vi "PCO_SetSoftFPS.vi"(0 "ph":u64, 1 "dwFPSin":u32, 2 "dwExp":u32, 3 "wTimeBaseExp":u16(ring) items=["ns", "us", "ms"], 4 "wFlags":u16, 5 "error in (no error)":errorcluster {"code" format="%x"}) -> (14 "ph_out":u64, 15 "ErrorMessage":i32 format="%x", 16 "dwFPSout":u32, 18 "wFlagsOut":u16, 19 "error out":errorcluster {"code" format="%x"})   [LabVIEW 2019, in "SDK.lvlib" / "TimingControl.lvlib"]
doc: "Setss the timing for the specified FPS (frames per second). The FPS is set by running an iterative loop, so reponse time may be slow."
uses:
  TimingControl.lvlib
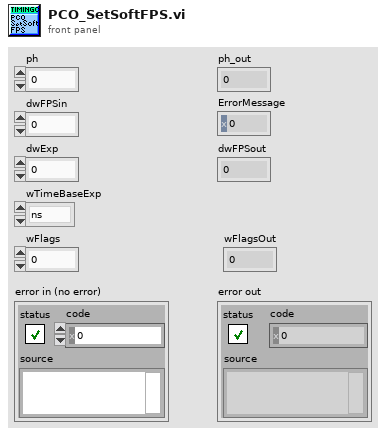
[diagram p1: front panel]
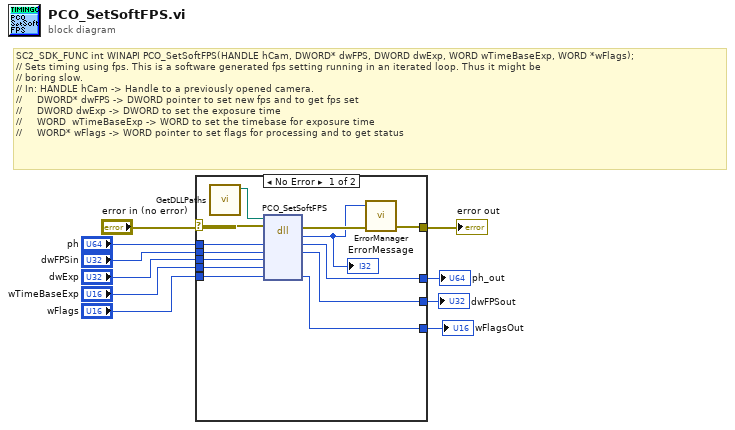
[diagram p0: block diagram]
diagram:
  # "SC2_SDK_FUNC int WINAPI PCO_SetSoftFPS(HANDLE hCam, DWORD* dwFPS, DWORD dwExp, WORD wTimeBaseExp, WORD *wFlags);\n// Sets timing using fps. This is a software generated fps setting running in an iterated loop. Thus it might be\n// boring slow.\n// In: HANDLE hCam -> Handle to a previously opened camera.\n//     DWORD* dwFPS -> DWORD pointer to set new fps and to get fps set\n//     DWORD dwExp -> DWORD to set the exposure time\n//     WORD  wTimeBaseExp -> WORD to set the timebase for exposure time\n//     WORD* wFlags -> WORD pointer to set flags for processing and to get status"
  n1 = case shown="No Error" "error in (no error)" {
    selector: "error in (no error)" -> [w21 w27]
    tunnel: "ph" -> [w23 w26]
    tunnel: "dwFPSin" -> [w22 w25]
    tunnel: [w19 w27] -> w9
    tunnel: [w16 w26] -> w7
    tunnel: [w15 w25] -> w6
    tunnel: "dwExp" -> [w14 _]
    tunnel: "wTimeBaseExp" -> [w13 _]
    tunnel: "wFlags" -> [w12 w24]
    tunnel: [w11 w24] -> w1
    frame No Error {
      n2 = call "GetDLLPaths.vi"() -> ("SC2_Cam_Path"=w17:path)  [unwired: 8 in, 3 out]
      n3 = dll-call lib="?" fn="PCO_SetSoftFPS"(path in=w17, error in=w21, "ph"=w23, "dwFPS"=w22, "dwExp"=w14, "wTimeBaseExp"=w13, "wFlags"=w12) -> (error out=w20:errorcluster, "return type"=w18:i32, "ph"=w16:u64, "dwFPS"=w15:u32, "wFlags"=w11:u16)  [unwired: 3 in, 1 out]
      "ErrorMessage" <- w18
      n4 = call "ErrorManager.vi"("error in (no error)"=w20, "error code"=w18) -> ("error out"=w19:errorcluster)  [unwired: 2 in, 1 out]
    }
    frame Error {
    }
  }
  "error out" <- w9
  "ph_out" <- w7
  "dwFPSout" <- w6
  "wFlagsOut" <- w1
